vi "Setupbearbeiten_interface.vi"(7 "VI Refnum":refnum<vi>, 8 "error in (no error)":errorcluster, 10 "Setup in":refnum<class "Setup.lvclass">, 11 "Daten":T1={"Report.lvclass"=refnum, "Norm"="", "last State"=enum."Initialize", "Norm ID"=0, "EMTestCWS500N.lvclass"=refnum, "CEG4500.lvclass"=refnum, "Tektronix RSA5106A.lvclass"=refnum, "erfolgreich"=FALSE, "Device Enum"=enum."emTestCWS500N", "Test Enum"=enum."ESD", "debug"=FALSE, "tab"=enum."Hauptmenü", "ESD Pistol.lvclass"=refnum, "SubPnl Refnum"=refnum, "TabCtl Refnum"=refnum, "ButtonsEinblenden?"=FALSE, "VKey"=enum."ASCII", "last Test"=refnum, "Class 4.lvclass"=refnum}) -> (0 "error out":errorcluster, 2 "Setup out":refnum<class "Setup.lvclass">, 3 "Abbrechen out":bool=TRUE)   [LabVIEW 2013, in "Dialogs.lvlib"]
uses:
  lib/Dialogs.lvlib
  Main/controls/Data.ctl
  classes/Datastructure/Report/Report.lvclass
  classes/Devices/emTestCWS500N/EMTestCWS500N.lvclass
  classes/Devices/CEG4500/CEG4500.lvclass
  classes/Devices/Tektronix RSA5106A/Tektronix RSA5106A.lvclass
  ESD Pistol.lvclass
  classes/Datastructure/Test/Test.lvclass
  classes/Devices/Class4/Class 4.lvclass
  Main/controls/State.ctl
  classes/Devices/DeviceInterface/Devices.ctl
  classes/Tests/TestInterface/Tests.ctl
  Tabs.ctl
  <vilib>/event_ctls.llb/eventvkey.ctl
  classes/Datastructure/Setup/Setup.lvclass
panel:
  in  "Setup in 2":refnum<class "Setup.lvclass">
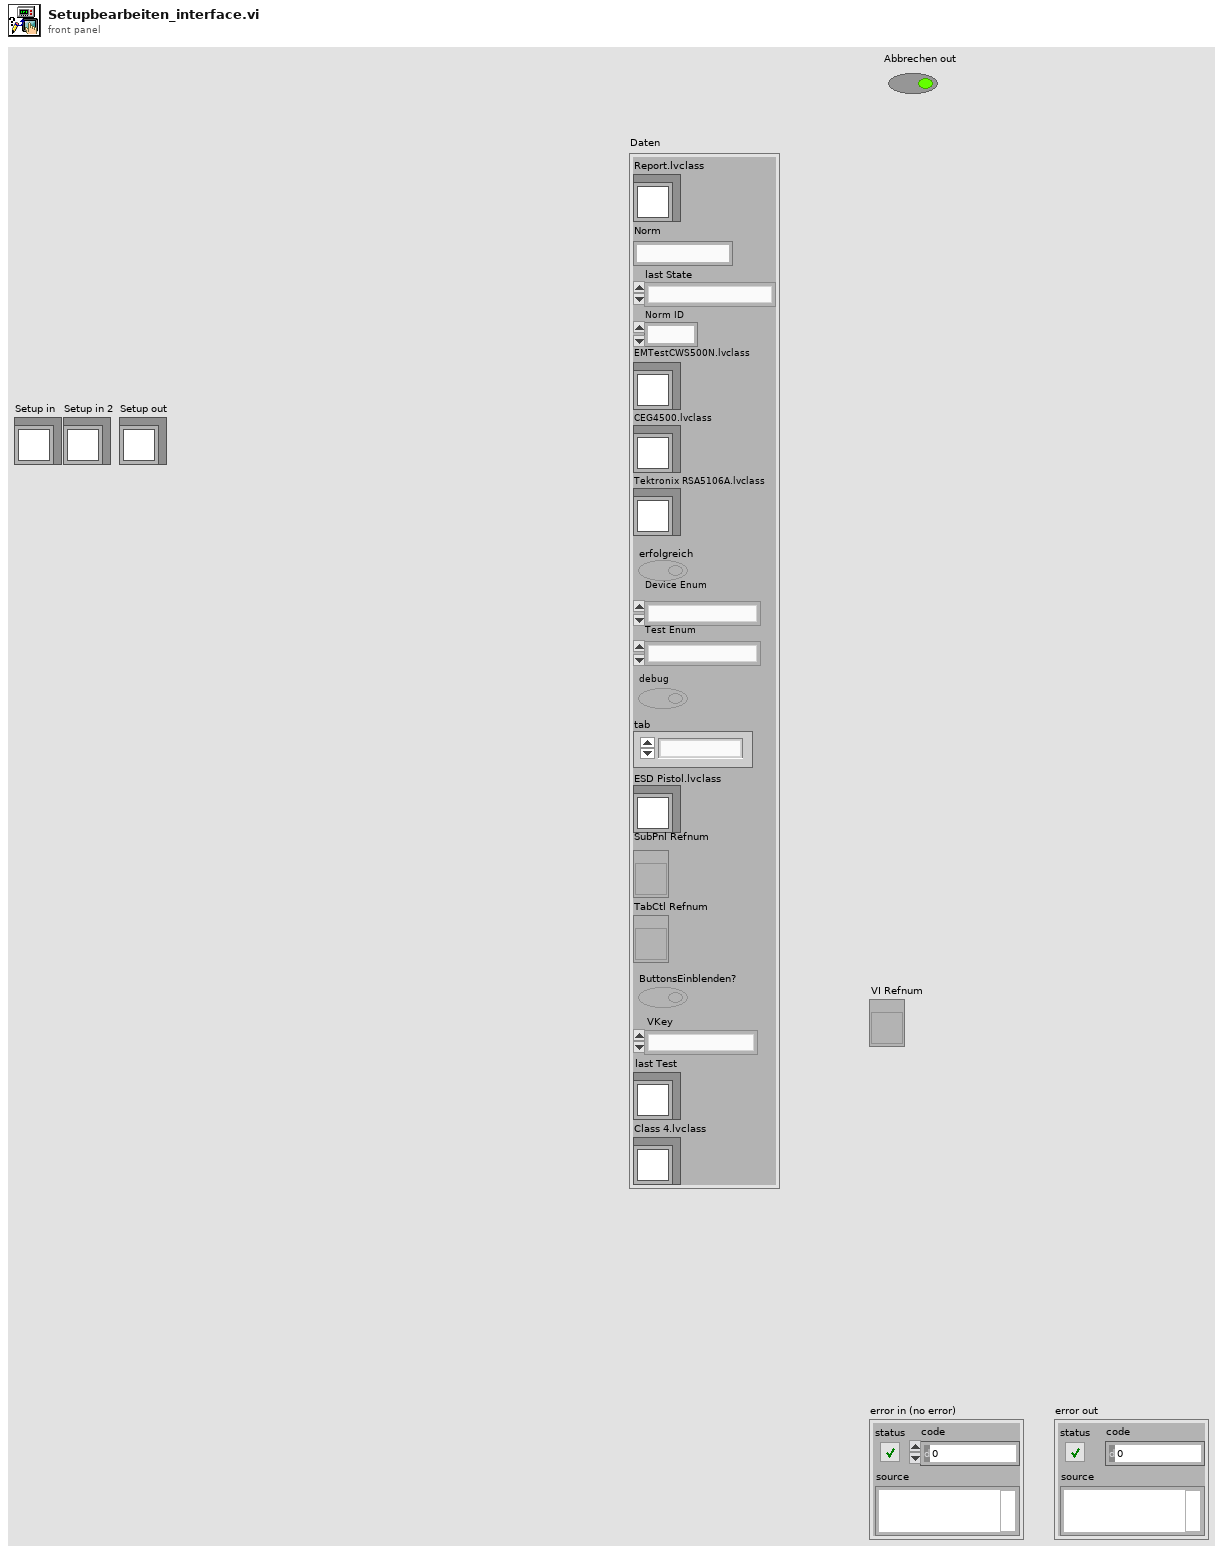
[diagram p1: front panel]
types:
  T1 = typedef "Data.ctl" = cluster{"Report.lvclass":refnum<class "Report.lvclass">, "Norm":string, "last State":T2, "Norm ID":i32, "EMTestCWS500N.lvclass":refnum<class "EMTestCWS500N.lvclass">, "CEG4500.lvclass":refnum<class "CEG4500.lvclass">, "Tektronix RSA5106A.lvclass":refnum<class "Tektronix RSA5106A.lvclass">, "erfolgreich":bool, "Device Enum":T3, "Test Enum":T4, "debug":bool, "tab":T5, "ESD Pistol.lvclass":refnum<class "ESD Pistol.lvclass">, "SubPnl Refnum":refnum<vi>, "TabCtl Refnum":refnum<vi>, "ButtonsEinblenden?":bool, "VKey":T6, "last Test":refnum<class "Test.lvclass">, "Class 4.lvclass":refnum<class "Class 4.lvclass">}
  T2 = typedef "State.ctl" = enum16{"create Pdf", "edit Report", "load Report", "save Report", "do Test", "CDN Kalibrierung", "enter Report Parameters", "new Test", "Protokoll", "read Tree", "update Tree", "Fehler", "Initialize", "Wait for Event", "Exit"}
  T3 = typedef "Devices.ctl" = enum16{"unbekannt", "ESD Pistol", "Tektronix RSA5106A", "emTestCWS500N", "CEG-4500"}
  T4 = typedef "Tests.ctl" = enum16{"unbekannt", "Störaussendung", "Burst", "ESD", "Surge", "Spannungseinbruch", "HF-Felder"}
  T5 = typedef "Tabs.ctl" = enum32{"Hauptmenü", "Prüfbericht", "Einstellungen"}
  T6 = typedef "eventvkey.ctl" = enum16{"ASCII", "Enter", "Return", "Shift", "Ctrl", "Alt", "Cmd", "Opt", "Caps", "NumLock", "Clear", "Break", "Up", "Down", "Left", "Right", "Insert", "Delete", "Home", "End", "PageUp", "PageDown", "Escape", "Help", "Pause", "ScrollLock", "F1", "F2", "F3", "F4", "F5", "F6", "F7", "F8", "F9", "F10", "F11", "F12", "F13", "F14", "F15", "F16", "F17", "F18", "F19", "F20", "F21", "F22", "F23", "F24", "Play", "VolumeUp", "VolumeDown", "Mute", "Two Byte Char"}
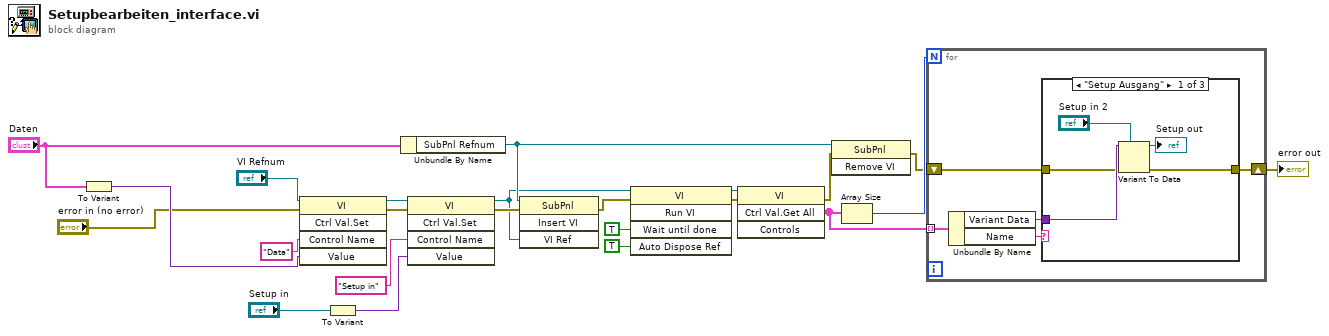
[diagram p0: block diagram]
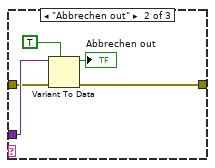
[diagram p2: hidden frame]
diagram:
  n1 = To Variant(anything="Daten") -> (Variant=w13:variant)
  n2 = invoke class="VI" method="Ctrl Val.Set"(reference="VI Refnum", error in="error in (no error)", "Control Name"="Data", "Value"=w13) -> (reference out=w9:refnum<vi>, error out=w8:errorcluster)  [unwired: 1 in, 3 out]
  n3 = To Variant(anything="Setup in") -> (Variant=w3:variant)
  n4 = Unbundle By Name("Daten") -> ("SubPnl Refnum"=w10:refnum<vi>)
  n5 = invoke class="VI" method="Ctrl Val.Set"(reference=w9, error in=w8, "Control Name"="Setup in", "Value"=w3) -> (reference out=w6:refnum<vi>, error out=w7:errorcluster)  [unwired: 1 in, 3 out]
  n6 = invoke on="Invoke Node" class="SubPnl" method="Insert VI"(reference=w10, error in=w7, "VI Ref"=w6) -> (error out=w21:errorcluster)  [unwired: 1 in, 3 out]
  n7 = invoke on="Methodenknoten" class="VI" method="Run VI"(reference=w6, error in=w21, "Wait until done"=TRUE ("Warten bis beendet"), "Auto Dispose Ref"=TRUE ("Referenz automatisch schließen")) -> (reference out=w23:refnum<vi>, error out=w22:errorcluster)  [unwired: 1 in, 3 out]
  n8 = invoke class="VI" method="Ctrl Val.Get All"(reference=w23, error in=w22) -> (error out=w16:errorcluster, "Get All Control Values Variant"=w18:cluster{"Name":string, "Variant Data":variant}[])  [unwired: 2 in, 2 out]
  n9 = invoke on="Invoke Node" class="SubPnl" method="Remove VI"(reference=w10, error in=w16) -> (error out=w15:errorcluster)  [unwired: 1 in, 2 out]
  n10 = Array Size(array=w18) -> (size(s)=w17:i32)
  n11 = for {
    N: w17 -> [_]
    tunnel: w18 -> [w28] mode=indexing
    shift-right: [w24] -> w14
    shift-left: w15 -> [w25]
    n12 = Unbundle By Name(w28) -> ("Variant Data"=w26:variant, "Name"=w27:string)
    n13 = case shown="\"Setup Ausgang\"" w27 {
      tunnel: w26 -> [w33 w38 _]
      tunnel: w25 -> [w32 w37 w39]
      tunnel: [w31 w36 w39] -> w24
      frame "Setup Ausgang" {
        n14 = Variant To Data(error in=w32, type="Setup in 2", Variant=w33) -> (data=→"Setup out":refnum<class "Setup.lvclass">, error out=w31:errorcluster)
      }
      frame "Abbrechen out" {
        n15 = Variant To Data(error in=w37, type=TRUE ("Boolean"), Variant=w38) -> (data=→"Abbrechen out":bool, error out=w36:errorcluster)
      }
      frame Default {
      }
    }
  }
  "error out" <- w14
